vi "KMAX initialize.vi"(8 "error in (no error)":errorcluster, 11 "Refnum in":T2) -> (0 "error out":errorcluster, 2 "New Image":T1, 3 "Refnum out":T2)   [LabVIEW 2023]
uses:
  <vilib>/userDefined/High Color/IMAQdx.ctl
  <vilib>/vision/Image Controls.llb/IMAQ Image.ctl
  <vilib>/vision/driver/NI_Vision_Acquisition_Software.lvlib
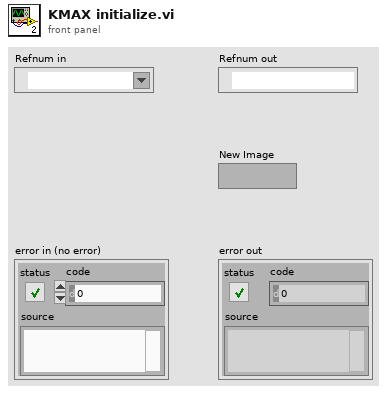
[diagram p1: front panel]
types:
  T1 = typedef "IMAQ Image.ctl" = refnum<image>
  T2 = typedef "IMAQdx.ctl" = refnum<k21>
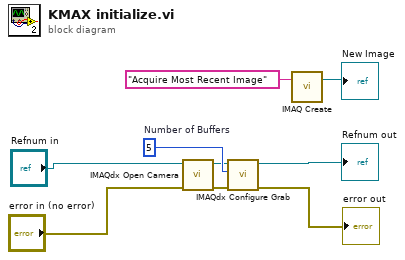
[diagram p0: block diagram]
diagram:
  w5 = u32 5  # Number of Buffers
  n1 = call <vilib>:"IMAQdx Open Camera.vi"("error in"="error in (no error)", "Session In"="Refnum in") -> ("error out"=w6:errorcluster, "Session Out"=w4:T2)  [unwired: 1 in, 7 out]
  n2 = call <vilib>:"IMAQdx Configure Grab.vi"("error in"=w6, "Number of Buffers"=w5, "Session In"=w4) -> ("error out"=→"error out":errorcluster, "Session Out"=→"Refnum out":T2)  [unwired: 7 in]
  n3 = call "IMAQ Create"("Image Name"="Acquire Most Recent Image") -> ("New Image"=→"New Image":T1)  [unwired: 3 in, 2 out]
